vi "PowerWrapper.vi"(10 "Power":dbl, 11 "DLLpath":path) -> (3 "DLLpathOUt":path)   [LabVIEW 2014]
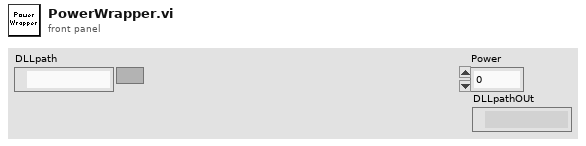
[diagram p1: front panel]
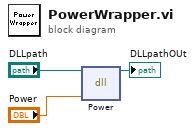
[diagram p0: block diagram]
diagram:
  n1 = dll-call lib="C:/Users/guss2/Desktop/GVI/Git/LVslicer/MachineController/DLL/MachineSimulator.dll" fn="Power"(path in="DLLpath", "Power"="Power") -> (path out=→"DLLpathOUt":path)  [unwired: 4 in, 1 out]
